vi "LVClass_CameraSet Get CameraParameter.vi"(0 "CameraSet in":refnum<class "CameraSet.lvclass">, 11 "error in (no error)":errorcluster) -> (4 "CameraSet out":refnum<class "CameraSet.lvclass">, 6 "ListOfGettableParameter":T1[](array[typedef]), 8 "ListOfGettableSettableParameter":T1[](array[typedef]), 15 "error out":errorcluster)   [LabVIEW 2020, in "CameraSet.lvclass"]
uses:
  CameraSet.lvclass
  CameraParametersSetup.ctl
  CameraParameters_Type.ctl
  ParameterID.ctl
  CameraParameters_Authorization.ctl
  CameraParameters_OnFlyAuthorization.ctl
  CameraSet.lvclass/CameraSet.ctl
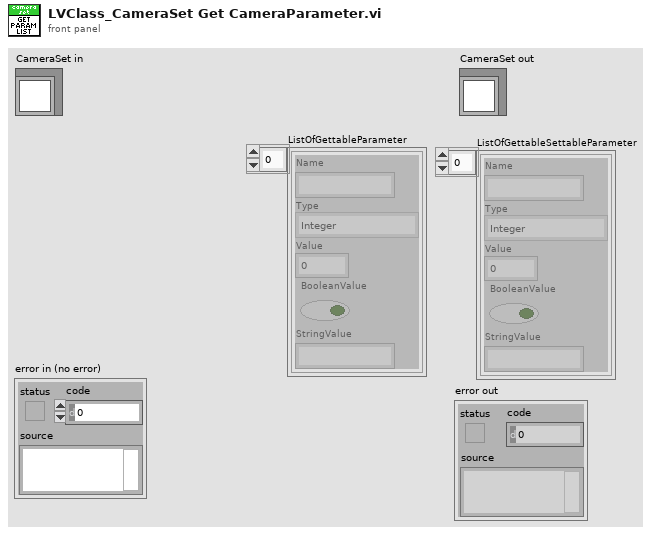
[diagram p1: front panel]
types:
  T1 = typedef "CameraParametersSetup.ctl" = cluster{"Name":string, "Type":T2, "Value":dbl, "BooleanValue":bool, "StringValue":string}
  T2 = typedef "CameraParameters_Type.ctl" = enum16{"Integer", "Real", "String", "Boolean"}
  T3 = typedef "CameraParameters_Authorization.ctl" = enum16{"Disable", "Gettable", "Settable - Gettable"}
  T4 = typedef "CameraParameters_OnFlyAuthorization.ctl" = enum16{"None", "Gettable", "Settable", "Settable - Gettable"}
  T5 = typedef "ParameterID.ctl" = cluster{"Name":string, "Type":T2, "Authorization":T3, "OnFlyAuthorization":T4, "StringDefault":string, "Default":dbl, "Min":dbl, "Max":dbl, "Boolean":bool, "StringParameterList":string[]}
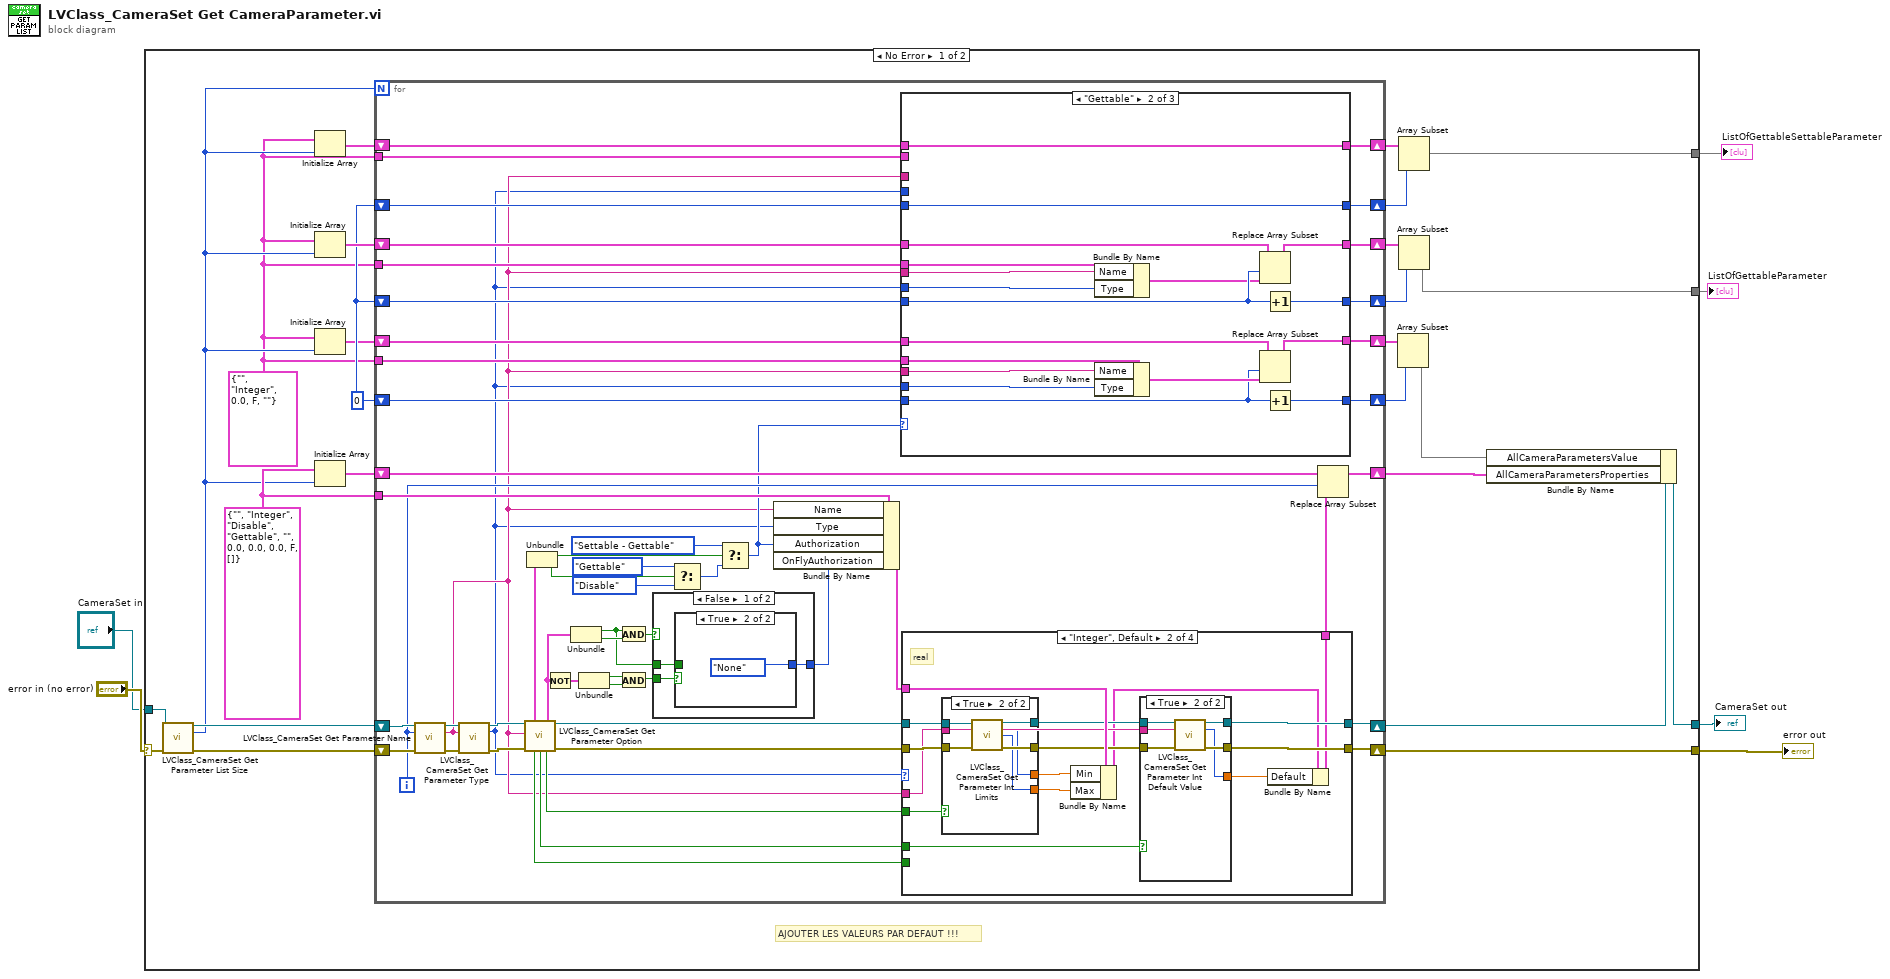
[diagram p0: block diagram]
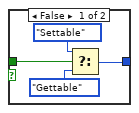
[diagram p2: hidden frame]
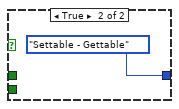
[diagram p3: hidden frame]
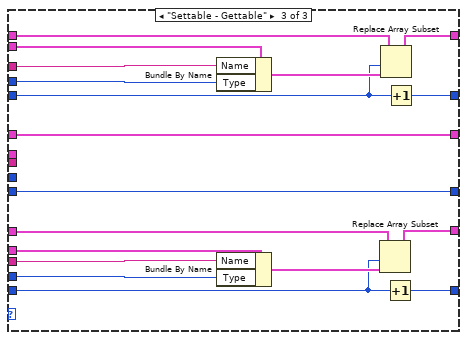
[diagram p5: hidden frame]
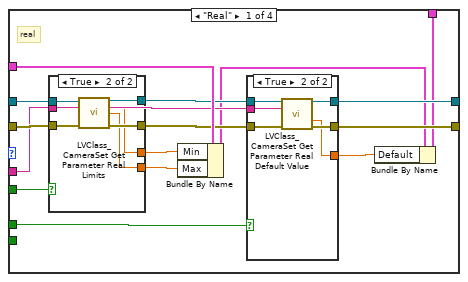
[diagram p6: hidden frame]
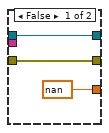
[diagram p7: hidden frame]
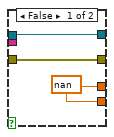
[diagram p8: hidden frame]
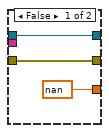
[diagram p9: hidden frame]
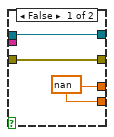
[diagram p10: hidden frame]
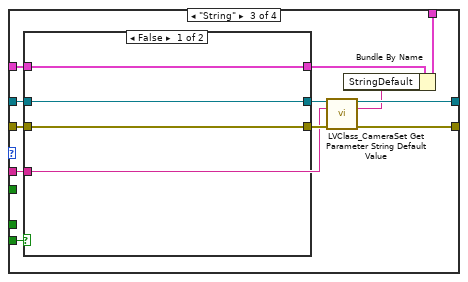
[diagram p11: hidden frame]
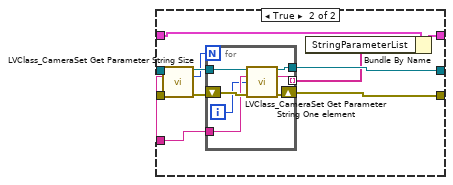
[diagram p12: hidden frame]
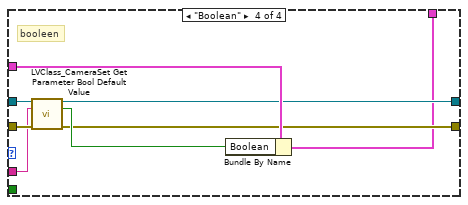
[diagram p13: hidden frame]
diagram:
  n1 = case shown="No Error" "error in (no error)" {
    selector: "error in (no error)" -> [w29 w246]
    tunnel: [w28 w246] -> w5
    tunnel: [w30 w245] -> w3
    tunnel: "CameraSet in" -> [w27 w245]
    tunnel: [w15 _] -> w2
    tunnel: [w14 _] -> w1
    frame No Error {
      w10 = T1 {"Name"="", "Type"=enum."Integer", "Value"=0.0, "BooleanValue"=FALSE, "StringValue"=""} ("CameraParametersSetup")
      w13 = 0
      w23 = T5 {"Name"="", "Type"=enum."Integer", "Authorization"=enum."Disable", "OnFlyAuthorization"=enum."Gettable", "StringDefault"="", "Default"=0.0, "Min"=0.0, "Max"=0.0, "Boolean"=FALSE, "StringParameterList"=[]} ("CameraParameters")
      # "AJOUTER LES VALEURS PAR DEFAUT !!!"
      n2 = call "LVClass_CameraSet Get Parameter List Size.vi"("CameraSet.lvclass"=w27, "error in (no error)"=w29) -> ("CameraSet.lvclass"=w26:refnum<class "CameraSet.lvclass">, "size"=w11:i32, "error out"=w31:errorcluster)  [unwired: 11 in]
      n3 = Initialize Array(w10, w11) -> (w18:T1[])
      n4 = Initialize Array(w10, w11) -> (w20:T1[])
      n5 = Initialize Array(w10, w11) -> (w12:T1[])
      n6 = Initialize Array(w23, w11) -> (w24:T5[])
      n7 = for {
        N: w11 -> [_]
        tunnel: w23 -> [w80]
        shift-right: [w79] -> w28
        shift-left: w31 -> [w83]
        shift-right: [w78] -> w25
        shift-left: w26 -> [w84]
        shift-right: [w66] -> w22
        shift-left: w24 -> [w67]
        shift-right: [w62] -> w19
        shift-left: w13 -> [w63]
        shift-right: [w61] -> w21
        shift-left: w20 -> [w59]
        tunnel: w10 -> [w58]
        tunnel: w10 -> [w55]
        shift-right: [w56] -> w17
        shift-left: w18 -> [w57]
        shift-right: [w53] -> w16
        shift-left: w13 -> [w54]
        shift-right: [w38] -> w8
        shift-left: w13 -> [w37]
        shift-right: [w35] -> w9
        shift-left: w12 -> [w36]
        tunnel: w10 -> [w34]
        i -> [w64]
        n8 = call "LVClass_CameraSet Get Parameter Name.vi"("CameraSet.lvclass"=w84, "index"=w64, "error in (no error)"=w83) -> ("CameraSet.lvclass"=w82:refnum<class "CameraSet.lvclass">, "parameter_name"=w33:string, "error out"=w81:errorcluster)  [unwired: 10 in]
        n9 = call "LVClass_CameraSet Get Parameter Type.vi"("CameraSet.lvclass"=w82, "parameter_name"=w33, "error in (no error)"=w81) -> ("CameraSet.lvclass"=w77:refnum<class "CameraSet.lvclass">, "Type"=w32:T2, "error out"=w76:errorcluster)  [unwired: 10 in]
        n10 = call "LVClass_CameraSet Get Parameter Option.vi"("CameraSet.lvclass"=w77, "parameter_name"=w33, "error in (no error)"=w76) -> ("Settable-Gettable?"=w50:cluster{"Settable":bool, "Gettable":bool}, "Settable-Gettable on fly?"=w43:cluster{"Settable":bool, "Gettable":bool}, "CameraSet.lvclass"=w75:refnum<class "CameraSet.lvclass">, "String enum"=w51:bool, "DefaultValueExist"=w52:bool, "minmax"=w68:bool, "error out"=w74:errorcluster)  [unwired: 6 in]
        n11 = Unbundle(w50) -> ("Settable"=w49:bool, "Gettable"=w48:bool)
        n12 = Not(x=w43) -> (.not. x?=w41:cluster{"Settable":bool, "Gettable":bool})
        n13 = Unbundle(w43) -> ("Settable"=w40:bool, "Gettable"=w47:bool)
        n14 = Unbundle(w41) -> ("Settable"=w42:bool, "Gettable"=w45:bool)
        n15 = And(x=w40, y=w47) -> (x .and. y?=w46:bool)
        n16 = And(x=w42, y=w45) -> (x .and. y?=w44:bool)
        n17 = case shown="False" w46 {
          tunnel: [w86 CameraParameters_OnFlyAuthorization."Settable - Gettable" ("OnFlyAuthorization")] -> w39
          tunnel: w44 -> [w87 _]
          tunnel: w40 -> [w85 _]
          frame False {
            n18 = case shown="True" w87 {
              tunnel: [w91 CameraParameters_OnFlyAuthorization."None" ("OnFlyAuthorization")] -> w86
              tunnel: w85 -> [w88 _]
              frame False {
                n19 = Select(t=CameraParameters_OnFlyAuthorization."Settable" ("OnFlyAuthorization"), s=w88, f=CameraParameters_OnFlyAuthorization."Gettable" ("OnFlyAuthorization")) -> (s? t:f=w91:T4)
              }
              frame True {
              }
            }
          }
          frame True {
          }
        }
        n20 = Select(t=CameraParameters_Authorization."Gettable" ("Authorization"), s=w48, f=CameraParameters_Authorization."Disable") -> (s? t:f=w71:T3)
        n21 = Select(t=CameraParameters_Authorization."Settable - Gettable", s=w49, f=w71) -> (s? t:f=w60:T3)
        n22 = Bundle By Name(cluster=w80, "Name"=w33, "Type"=w32, "Authorization"=w60, "OnFlyAuthorization"=w39) -> (w69:T5)
        n23 = case shown="\"Gettable\"" w60 {
          tunnel: w63 -> [w98 w117 w126]
          tunnel: [w98 w116 w126] -> w62
          tunnel: [w99 w115 w127] -> w61
          tunnel: w33 -> [_ w102 _]
          tunnel: w32 -> [_ w114 _]
          tunnel: w59 -> [w99 w112 w127]
          tunnel: w58 -> [_ w111 _]
          tunnel: w57 -> [w97 w109 w134]
          tunnel: [w97 w109 w133] -> w56
          tunnel: w33 -> [_ _ w132]
          tunnel: w32 -> [_ _ w131]
          tunnel: w55 -> [_ _ w130]
          tunnel: w54 -> [w96 w110 w129]
          tunnel: [w96 w110 w128] -> w53
          tunnel: [w94 w107 w118] -> w38
          tunnel: w37 -> [w94 w106 w119]
          tunnel: w36 -> [w95 w105 w124]
          tunnel: [w95 w104 w123] -> w35
          tunnel: w34 -> [_ w103 w120]
          tunnel: w33 -> [_ w101 w122]
          tunnel: w32 -> [_ w100 w121]
          frame "Disable", Default {
          }
          frame "Gettable" {
            n24 = Bundle By Name(cluster=w111, "Name"=w102, "Type"=w114) -> (w113:T1)
            n25 = Bundle By Name(cluster=w103, "Name"=w101, "Type"=w100) -> (w108:T1)
            n26 = Replace Array Subset(array=w112, new element=w113, index=w117) -> (w115:T1[])
            n27 = Replace Array Subset(array=w105, new element=w108, index=w106) -> (w104:T1[])
            n28 = Increment(x=w117) -> (x+1=w116:i32)
            n29 = Increment(x=w106) -> (x+1=w107:i32)
          }
          frame "Settable - Gettable" {
            n30 = Bundle By Name(cluster=w130, "Name"=w132, "Type"=w131) -> (w135:T1)
            n31 = Bundle By Name(cluster=w120, "Name"=w122, "Type"=w121) -> (w125:T1)
            n32 = Replace Array Subset(array=w124, new element=w125, index=w119) -> (w123:T1[])
            n33 = Replace Array Subset(array=w134, new element=w135, index=w129) -> (w133:T1[])
            n34 = Increment(x=w119) -> (x+1=w118:i32)
            n35 = Increment(x=w129) -> (x+1=w128:i32)
          }
        }
        n36 = case shown="\"Integer\", Default" w32 {
          tunnel: w69 -> [w150 w184 w207 w243]
          tunnel: w33 -> [w144 w178 w209 w240]
          tunnel: [w141 w175 w211 w238] -> w79
          tunnel: w75 -> [w149 w183 w215 w242]
          tunnel: w74 -> [w148 w182 w214 w241]
          tunnel: [w140 w174 w212 w239] -> w78
          tunnel: w52 -> [w136 w170 _ _]
          tunnel: w68 -> [w147 w181 _ _]
          tunnel: w51 -> [_ _ w205 _]
          tunnel: [w138 w172 w204 w237] -> w65
          frame "Real" {
            # "real"
            n37 = case shown="True" w147 {
              tunnel: w144 -> [_ w169]
              tunnel: [w162 w168] -> w142
              tunnel: [w161 w167] -> w143
              tunnel: w149 -> [w161 w166]
              tunnel: w148 -> [w162 w165]
              tunnel: [w160 w164] -> w146
              tunnel: [w160 w163] -> w145
              frame False {
                w160 = nan ("f")
              }
              frame True {
                n38 = call "LVClass_CameraSet Get Parameter Real Limits.vi"("CameraSet.lvclass"=w166, "parameter_name"=w169, "error in (no error)"=w165) -> ("CameraSet.lvclass"=w167:refnum<class "CameraSet.lvclass">, "min"=w164:dbl, "max"=w163:dbl, "error out"=w168:errorcluster)  [unwired: 9 in]
              }
            }
            n39 = Bundle By Name(cluster=w150, "Min"=w146, "Max"=w145) -> (w139:T5)
            n40 = case shown="True" w136 {
              tunnel: w144 -> [_ w159]
              tunnel: w143 -> [w153 w158]
              tunnel: w142 -> [w152 w157]
              tunnel: [w152 w156] -> w141
              tunnel: [w153 w155] -> w140
              tunnel: [nan ("f") w154] -> w137
              frame False {
              }
              frame True {
                n41 = call "LVClass_CameraSet Get Parameter Real Default Value.vi"("CameraSet.lvclass"=w158, "parameter_name"=w159, "error in (no error)"=w157) -> ("CameraSet.lvclass"=w155:refnum<class "CameraSet.lvclass">, "defaultValue"=w154:dbl, "error out"=w156:errorcluster)  [unwired: 10 in]
              }
            }
            n42 = Bundle By Name(cluster=w139, "Default"=w137) -> (w138:T5)
          }
          frame "Integer", Default {
            # "real"
            n43 = case shown="True" w181 {
              tunnel: w178 -> [_ w203]
              tunnel: [w196 w202] -> w176
              tunnel: [w195 w201] -> w177
              tunnel: w183 -> [w195 w200]
              tunnel: w182 -> [w196 w199]
              tunnel: [w194 w198] -> w180
              tunnel: [w194 w197] -> w179
              frame False {
                w194 = nan ("f")
              }
              frame True {
                n44 = call "LVClass_CameraSet Get Parameter Int Limits.vi"("CameraSet.lvclass"=w200, "parameter_name"=w203, "error in (no error)"=w199) -> ("CameraSet.lvclass"=w201:refnum<class "CameraSet.lvclass">, "min"=w198:i32, "max"=w197:i32, "error out"=w202:errorcluster)  [unwired: 9 in]
              }
            }
            n45 = Bundle By Name(cluster=w184, "Min"=w180, "Max"=w179) -> (w173:T5)
            n46 = case shown="True" w170 {
              tunnel: w178 -> [_ w193]
              tunnel: w177 -> [w187 w192]
              tunnel: w176 -> [w186 w191]
              tunnel: [w186 w190] -> w175
              tunnel: [w187 w189] -> w174
              tunnel: [nan ("f") w188] -> w171
              frame False {
              }
              frame True {
                n47 = call "LVClass_CameraSet Get Parameter Int Default Value.vi"("CameraSet.lvclass"=w192, "parameter_name"=w193, "error in (no error)"=w191) -> ("CameraSet.lvclass"=w189:refnum<class "CameraSet.lvclass">, "Default value"=w188:i32, "error out"=w190:errorcluster)  [unwired: 10 in]
              }
            }
            n48 = Bundle By Name(cluster=w173, "Default"=w171) -> (w172:T5)
          }
          frame "String" {
            n49 = case shown="False" w205 {
              tunnel: w215 -> [w218 w229]
              tunnel: w214 -> [w217 w228]
              tunnel: [w218 w224] -> w213
              tunnel: [w217 w223] -> w210
              tunnel: w209 -> [_ w222]
              tunnel: w207 -> [w216 w221]
              tunnel: [w216 w219] -> w206
              frame False {
              }
              frame True {
                n50 = call "LVClass_CameraSet Get Parameter String Size.vi"("CameraSet.lvclass"=w229, "parameter name"=w222, "error in (no error)"=w228) -> ("CameraSet.lvclass"=w227:refnum<class "CameraSet.lvclass">, "size"=w225:i32, "error out"=w226:errorcluster)  [unwired: 10 in]
                n51 = for {
                  N: w225 -> [_]
                  tunnel: w222 -> [w234]
                  tunnel: [w231] -> w224
                  tunnel: w227 -> [w236]
                  shift-right: [w230] -> w223
                  shift-left: w226 -> [w235]
                  tunnel: [w232] -> w220 mode=indexing
                  i -> [w233]
                  n52 = call "LVClass_CameraSet Get Parameter String One element.vi"("CameraSet.lvclass"=w236, "parameter name"=w234, "index"=w233, "error in (no error)"=w235) -> ("CameraSet.lvclass"=w231:refnum<class "CameraSet.lvclass">, "value"=w232:string, "error out"=w230:errorcluster)  [unwired: 9 in]
                }
                n53 = Bundle By Name(cluster=w221, "StringParameterList"=w220) -> (w219:T5)
              }
            }
            n54 = call "LVClass_CameraSet Get Parameter String Default Value.vi"("CameraSet.lvclass"=w213, "parameter name"=w209, "error in (no error)"=w210) -> ("CameraSet.lvclass"=w212:refnum<class "CameraSet.lvclass">, "Default value"=w208:string, "error out"=w211:errorcluster)  [unwired: 10 in]
            n55 = Bundle By Name(cluster=w206, "StringDefault"=w208) -> (w204:T5)
          }
          frame "Boolean" {
            # "booleen"
            n56 = call "LVClass_CameraSet Get Parameter Bool Default Value.vi"("CameraSet.lvclass"=w242, "parameter_name"=w240, "error in (no error)"=w241) -> ("CameraSet.lvclass"=w239:refnum<class "CameraSet.lvclass">, "Default value"=w244:bool, "error out"=w238:errorcluster)  [unwired: 10 in]
            n57 = Bundle By Name(cluster=w243, "Boolean"=w244) -> (w237:T5)
          }
        }
        n58 = Replace Array Subset(array=w67, new element=w65, index=w64) -> (w66:T5[])
      }
      n59 = Array Subset(array=w9, length=w8) -> (w7:T1[])  [unwired: 1 in]
      n60 = Array Subset(array=w17, length=w16) -> (w14:T1[])  [unwired: 1 in]
      n61 = Array Subset(array=w21, length=w19) -> (w15:T1[])  [unwired: 1 in]
      n62 = Bundle By Name(cluster=w25, "AllCameraParametersValue"=w7, "AllCameraParametersProperties"=w22) -> (w30:refnum<class "CameraSet.lvclass">)
    }
    frame Error {
    }
  }
  "error out" <- w5
  "CameraSet out" <- w3
  "ListOfGettableParameter" <- w2
  "ListOfGettableSettableParameter" <- w1
